vi "WinPositioner_v17.vi"(4 "Reverse":bool=TRUE, 5 "Bring To Front? (Y)":bool, 6 "Display (1, 2...)":u8=1 caption="Display?", 7 "Hide/Show (Show)":bool=TRUE, 9 "Cluster":T1={"Xoffset"=1280.0, "Yoffset 2"=0.0, "X position"=2.7955271565495208, "Y position"=-0.5284552845528454, "Fine X position"=-0.20766773162939334, "Fine Y position"=-0.5060728744939267} {"X position" scale=0.0..10.0; "Fine X position" scale=0.0..10.0; "Y position" scale=0.0..10.0; "Fine Y position" scale=0.0..10.0}, 11 "Image":T2=refnum) -> (1 "Y position":dbl=1308.953128600112, 2 "X position":dbl=1141.2619808306708, 3 "CGH_x":T2(plugin-control))   [LabVIEW 2023]
uses:
  <vilib>/vision/Image Controls.llb/IMAQ Image.ctl
panel:
  out "output cluster":cluster{i32, i32}={1141, 1309}
  # "1"
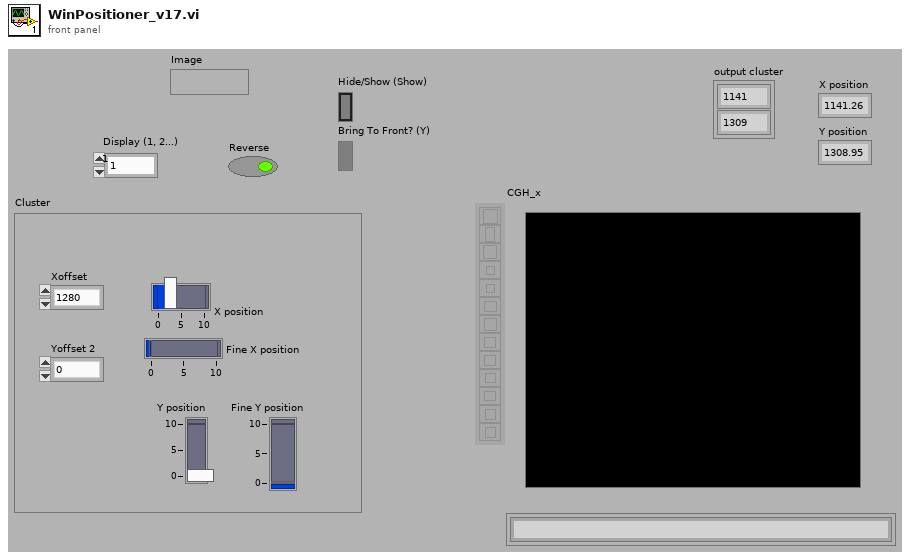
[diagram p1: front panel]
types:
  T1 = cluster{"Xoffset":dbl, "Yoffset 2":dbl, "X position":dbl, "Y position":dbl, "Fine X position":dbl, "Fine Y position":dbl}
  T2 = typedef "IMAQ Image.ctl" = refnum<image>
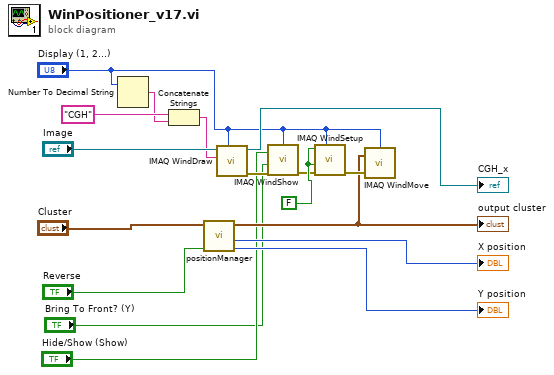
[diagram p0: block diagram]
diagram:
  w17 = FALSE
  n1 = Number To Decimal String(number="Display (1, 2...)") -> (decimal integer string=w2:string)  [unwired: 1 in]
  n2 = Concatenate Strings("CGH" ("Title"), w2) -> (w3:string)
  n3 = call "positionManager.vi"("just calculate"="Reverse", "Cluster"="Cluster") -> ("Y position out"=→"Y position":i32, "X position out"=→"X position":i32, "output cluster"=w8:cluster{i32, i32})  [unwired: 5 in]
  "output cluster" <- w8
  n4 = call "IMAQ WindDraw"("Window Number (0...15)"="Display (1, 2...)", "Title"=w3, "Image"="Image") -> ("error out"=w14:errorcluster, "Image Out (duplicate)"=→"CGH_x":T2)  [unwired: 7 in]
  n5 = call "IMAQ WindShow"("error in (no error)"=w14, "Bring To Front? (N)"="Bring To Front? (Y)", "Hide/Show (Show)"="Hide/Show (Show)", "Window Number (0...15)"="Display (1, 2...)") -> ("error out"=w15:errorcluster)  [unwired: 2 in, 2 out]
  n6 = call "IMAQ WindSetup"("Window Number (0...15)"="Display (1, 2...)", "error in (no error)"=w15, "Window has title bar? (Yes)"=w17, "Window can grow? (Yes)"=w17) -> ("error out"=w16:errorcluster)  [unwired: 7 in]
  n7 = call "IMAQ WindMove"("Window Number (0...15)"="Display (1, 2...)", "Coordinates (screen)"=w8, "error in (no error)"=w16) -> ()  [unwired: 2 in, 2 out]
